vi "Create Evaluations.vi"(8 "error in (no error)":errorcluster, 11 "IEvaluation in":refnum<class "GSM_ORFS_Custom.lvclass">) -> (0 "error out":errorcluster, 2 "Evaluations Out":T1[](array[typedef]) {"Low Limit" format="%#_13g"; "SI Scaling" items=["femto"=-15, "pico"=-12, "nano"=-9, "micro"=-6, "milli"=-3, "percent"=-2, ""=0, "kilo"=3, "mega"=6, "giga"=9, "tera"=12]}, 3 "IEvaluation out":refnum<class "GSM_ORFS_Custom.lvclass">)   [LabVIEW 2016, in "SeqAuto Evaluations.lvlib" / "GSM_ORFS_Custom.lvclass"]
uses:
  GSM_ORFS_Custom.lvclass
  C:/STS/Common/1.0/Sequence Automation/Plugins/SeqAuto IEvaluation.lvlibp/SeqAuto IEvaluation.lvclass
  Plugins/TestStand API Tools (TSAT).lvlibp/Evaluation Actions/Includes/Controls/TSAT Evaluation.ctl
  Plugins/TestStand API Tools (TSAT).lvlibp/Evaluation Actions/Includes/Controls/TSAT Eval SI Unit Scaling.ctl
  Plugins/TestStand API Tools (TSAT).lvlibp/Evaluation Actions/Includes/Controls/TSAT Evaluation Type.ctl
  GSM_ORFS_Custom.lvclass/GSM_ORFS_Custom.ctl
  Plugins/SeqAuto IEvaluation.lvlibp/Read Measurement Name.vi
  Plugins/TestStand API Tools (TSAT).lvlibp/Evaluation Actions/TSAT Evaluation Actions.lvlib
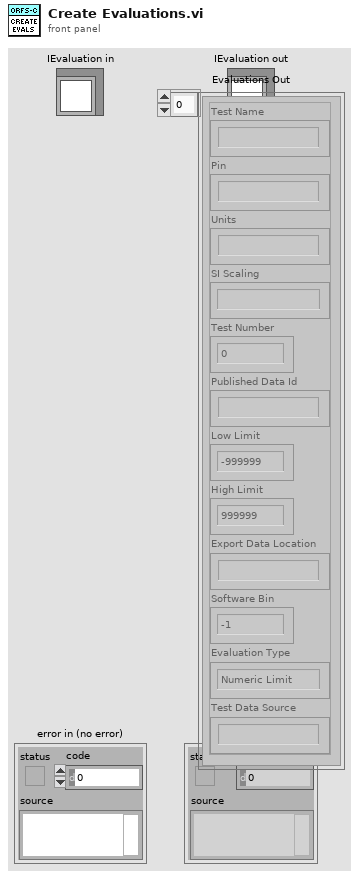
[diagram p1: front panel]
types:
  T1 = typedef "TestStand API Tools (TSAT).lvlibp/TSAT Evaluation Actions.lvlib/TSAT Evaluation.ctl" = cluster{"Test Name":string, "Pin":string, "Units":string, "SI Scaling":T2, "Test Number":i32, "Published Data Id":string, "Low Limit":dbl, "High Limit":dbl, "Export Data Location":string, "Software Bin":i64, "Evaluation Type":T3, "Test Data Source":string}
  T2 = typedef "TestStand API Tools (TSAT).lvlibp/TSAT Evaluation Actions.lvlib/TSAT Eval SI Unit Scaling.ctl" = i16
  T3 = typedef "TestStand API Tools (TSAT).lvlibp/TSAT Evaluation Actions.lvlib/TSAT Evaluation Type.ctl" = enum16{"Numeric Limit", "Pass/Fail", "None"}
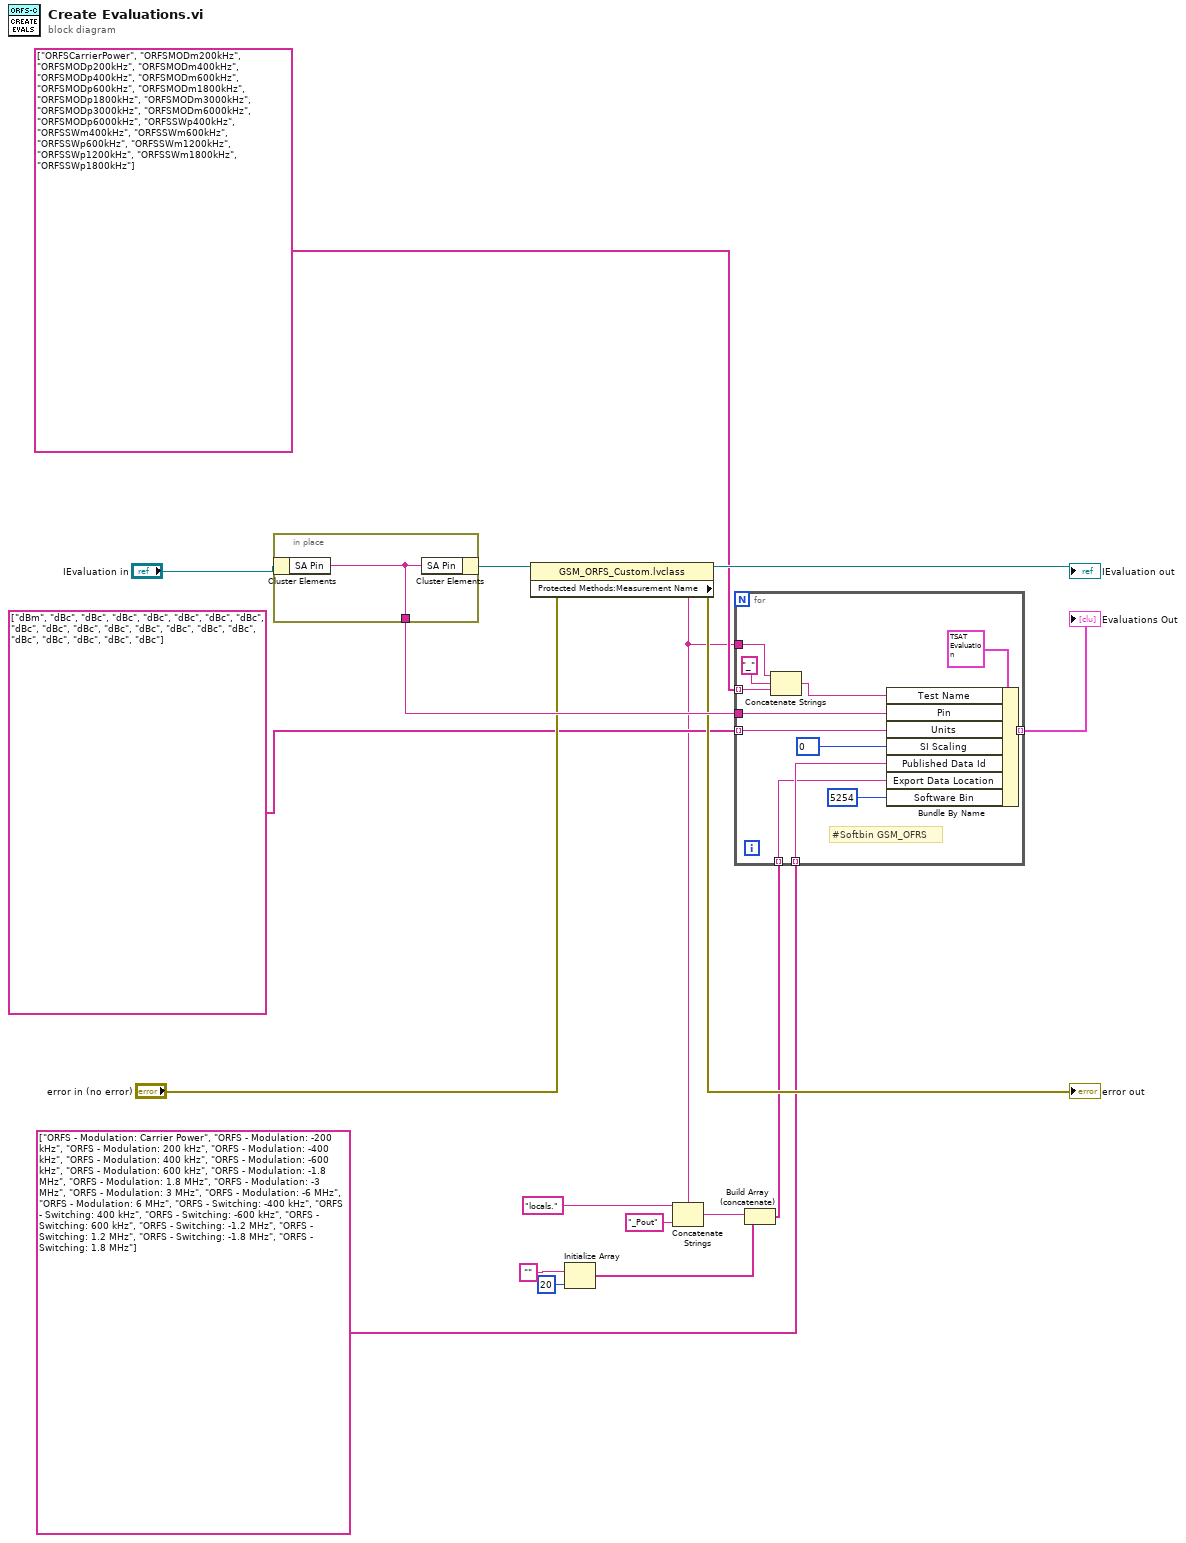
[diagram p0: block diagram]
diagram:
  n1 = in-place {
    in-place-border: [w19] -> w17
    n2 = in-place-cluster #1("IEvaluation in") -> ("SA Pin"=w19:string)
    n3 = in-place-cluster #1("SA Pin"=w19) -> (w18:refnum<class "GSM_ORFS_Custom.lvclass">)
  }
  n4 = property class="GSM_ORFS_Custom.lvclass"(reference=w18, error in="error in (no error)") -> (reference out=→"IEvaluation out":refnum<class "GSM_ORFS_Custom.lvclass">, error out=→"error out":errorcluster, "Protected Methods:Measurement Name"=w2:string)
  n5 = Initialize Array("" ("PublishedDataID"), 20 ("dimension size")) -> (w3:string[])
  n6 = Concatenate Strings("locals." ("PublishedDataID"), w2, "_Pout" ("string")) -> (w4:string)
  n7 = Build Array (concatenate)(w4, w3) -> (w1:string[])
  n8 = for {
    tunnel: w17 -> [w30]
    tunnel: [w28] -> w14 mode=indexing
    tunnel: w2 -> [w26]
    tunnel: string[] ["ORFSCarrierPower", "ORFSMODm200kHz", "ORFSMODp200kHz", "ORFSMODm400kHz", "ORFSMODp400kHz", "ORFSMODm600kHz", "ORFSMODp600kHz", "ORFSMODm1800kHz", "ORFSMODp1800kHz", "ORFSMODm3000kHz", "ORFSMODp3000kHz", "ORFSMODm6000kHz", "ORFSMODp6000kHz", "ORFSSWp400kHz", "ORFSSWm400kHz", "ORFSSWm600kHz", "ORFSSWp600kHz", "ORFSSWm1200kHz", "ORFSSWp1200kHz", "ORFSSWm1800kHz", "ORFSSWp1800kHz"] -> [w25] mode=indexing
    tunnel: string[] ["dBm", "dBc", "dBc", "dBc", "dBc", "dBc", "dBc", "dBc", "dBc", "dBc", "dBc", "dBc", "dBc", "dBc", "dBc", "dBc", "dBc", "dBc", "dBc", "dBc", "dBc"] -> [w24] mode=indexing
    tunnel: string[] ["ORFS - Modulation: Carrier Power", "ORFS - Modulation: -200 kHz", "ORFS - Modulation: 200 kHz", "ORFS - Modulation: -400 kHz", "ORFS - Modulation: 400 kHz", "ORFS - Modulation: -600 kHz", "ORFS - Modulation: 600 kHz", "ORFS - Modulation: -1.8 MHz", "ORFS - Modulation: 1.8 MHz", "ORFS - Modulation: -3 MHz", "ORFS - Modulation: 3 MHz", "ORFS - Modulation: -6 MHz", "ORFS - Modulation: 6 MHz", "ORFS - Switching: -400 kHz", "ORFS - Switching: 400 kHz", "ORFS - Switching: -600 kHz", "ORFS - Switching: 600 kHz", "ORFS - Switching: -1.2 MHz", "ORFS - Switching: 1.2 MHz", "ORFS - Switching: -1.8 MHz", "ORFS - Switching: 1.8 MHz"] -> [w23] mode=indexing
    tunnel: w1 -> [w21] mode=indexing
    w29 = T2 0 items=["femto"=-15, "pico"=-12, "nano"=-9, "micro"=-6, "milli"=-3, "percent"=-2, ""=0, "kilo"=3, "mega"=6, "giga"=9, "tera"=12] ("SI Scaling")
    # "#Softbin GSM_OFRS"
    n9 = Concatenate Strings(w26, "_" ("string"), w25) -> (w27:string)
    n10 = Bundle By Name(cluster=T1 {"Test Name"="", "Pin"="", "Units"="", "SI Scaling"=0, "Test Number"=0, "Published Data Id"="", "Low Limit"=-999999.0, "High Limit"=999999.0, "Export Data Location"="", "Software Bin"=-1, "Evaluation Type"=enum."Numeric Limit", "Test Data Source"=""} ("Evaluation"), "Test Name"=w27, "Pin"=w30, "Units"=w24, "SI Scaling"=w29, "Published Data Id"=w23, "Export Data Location"=w21, "Software Bin"=i64 5254) -> (w28:T1)
  }
  "Evaluations Out" <- w14
